vi "readDataArray.vi"(8 "error in (no error)":errorcluster, 10 "array":string[][](array[string]), 11 "Ao8FileReader in":refnum<class "Ao8FileReader.lvclass">) -> (0 "error out":errorcluster, 3 "Ao8FileReader out":refnum<class "Ao8FileReader.lvclass">)   [LabVIEW 2011, in "Tools.lvlib" / "Filing.lvlib" / "Ao8FileReader.lvclass"]
uses:
  Ao8FileReader.lvclass
  Ao8FileReader.lvclass/Ao8FileReader.ctl
  Hal/Channels/VoltOutput/AnalogOutput.lvclass
panel:
  out "channelAddresses":string[](array[string])
  out "Defaults":dbl[](array[numeric])
  out "data":dbl[][](array[numeric])
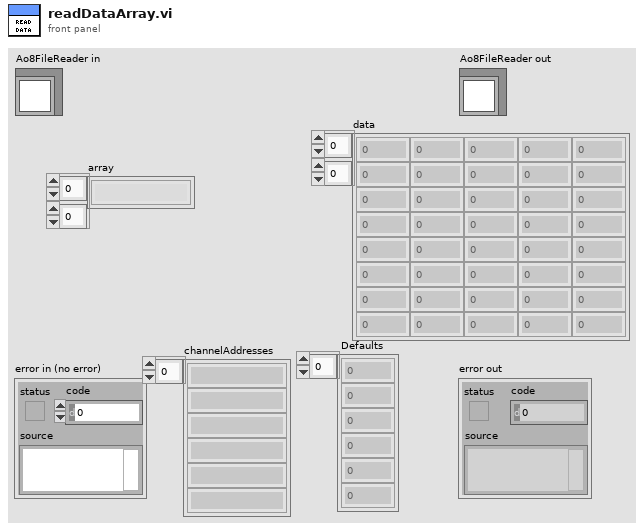
[diagram p1: front panel]
types:
  T1 = cluster{"Clock source":string, "Clock rate":dbl, "Start trigger line":string, "Sample Rate":dbl, "Sample No.":dbl}
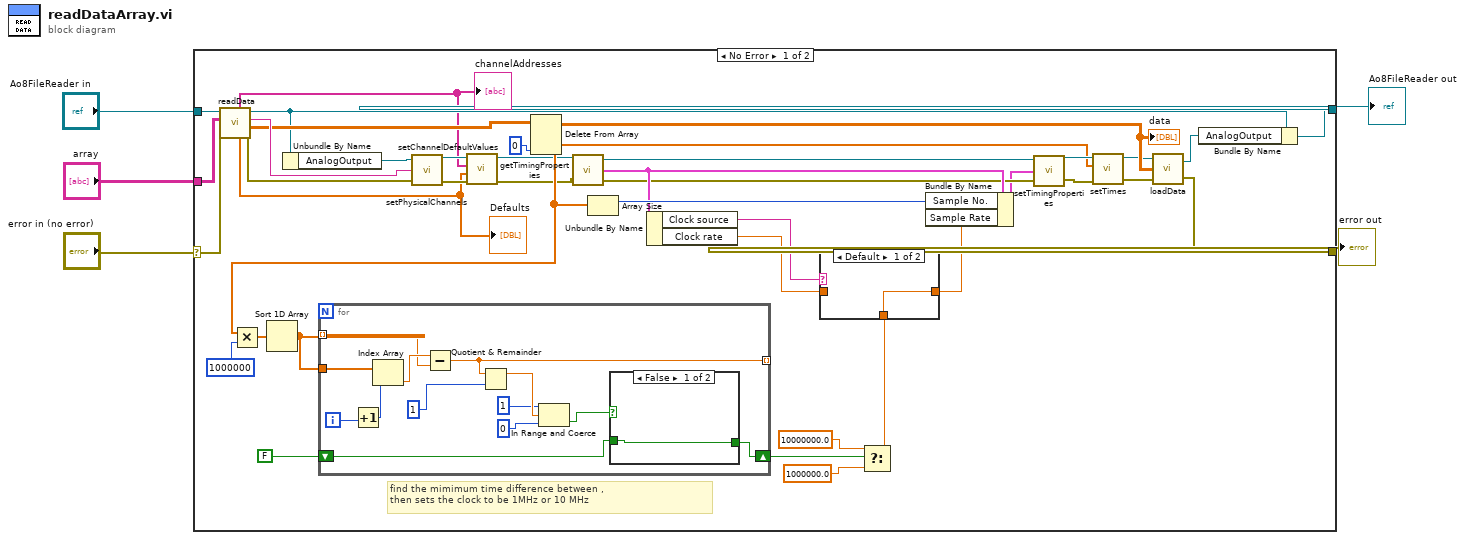
[diagram p0: block diagram]
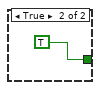
[diagram p3: hidden frame]
diagram:
  n1 = case shown="No Error" "error in (no error)" {
    selector: "error in (no error)" -> [w43 w63]
    tunnel: "Ao8FileReader in" -> [w45 w64]
    tunnel: "array" -> [w44 _]
    tunnel: [w13 w64] -> w3
    tunnel: [w16 w63] -> w2
    frame No Error {
      # "find the mimimum time difference between ,\nthen sets the clock to be 1MHz or 10 MHz"
      n2 = call-dynamic "readData.vi"("error in (no error)"=w43, "array"=w44, "FileReader in"=w45) -> ("error out"=w40:errorcluster, "Array"=w23:dbl[][], "channels"=w41:string, "FileReader out"=w15:refnum<class "Ao8FileReader.lvclass">, "Defaults"=w6:dbl[], "channelAddresses"=w7:string[])  [unwired: 3 in]
      "Defaults" <- w6
      "channelAddresses" <- w7
      n3 = Unbundle By Name(w15) -> ("AnalogOutput"=w42:refnum<class "AnalogOutput.lvclass">)
      n4 = call-dynamic "setPhysicalChannels.vi"("error in (no error)"=w40, "Physical Channels"=w41, "AnalogOutput.lvclass in"=w42) -> ("error out"=w10:errorcluster, "AnalogOutput.lvclass out"=w11:refnum<class "AnalogOutput.lvclass">)
      n5 = call "setChannelDefaultValues.vi"("error in (no error)"=w10, "calibratedValues"=w6, "channel_addresses"=w7, "AnalogOutput in"=w11) -> ("error out"=w9:errorcluster, "AnalogOutput out"=w8:refnum<class "AnalogOutput.lvclass">)  [unwired: 6 in]
      n6 = Delete From Array(array=w23, index (col)=0 ("disabled index (col)")) -> (deleted portion=w12:dbl[], array with subset deleted=w21:dbl[][])  [unwired: 2 in]
      "data" <- w21
      n7 = Multiply(x=w12, y=1000000) -> (x*y=w33:dbl[])
      n8 = Sort 1D Array(array=w33) -> (sorted array=w38:dbl[])
      n9 = for {
        tunnel: w38 -> [w56] mode=indexing
        tunnel: w38 -> [w60]
        tunnel: [w51] -> _ mode=indexing
        shift-right: [w48] -> w36
        shift-left: FALSE -> [w49]
        i -> [w59]
        n10 = Increment(x=w59) -> (x+1=w58:i32)
        n11 = Index Array(array=w60, index=w58) -> (element=w57:dbl)
        n12 = Subtract(x=w57, y=w56) -> (x-y=w51:dbl)
        n13 = Quotient & Remainder(x=w51, y=1) -> (x-y*floor(x/y)=w54:dbl)  [unwired: 1 out]
        n14 = In Range and Coerce(upper limit=1, x=w54, lower limit=0) -> (In Range?=w50:bool)  [unwired: 1 out]
        n15 = case shown="False" w50 {
          tunnel: w49 -> [w61 _]
          tunnel: [w61 TRUE] -> w48
          frame False {
          }
          frame True {
          }
        }
      }
      n16 = call "getTimingProperties.vi"("AnalogOutput.lvclass in"=w8, "error in (no error)"=w9) -> ("AnalogOutput.lvclass out"=w26:refnum<class "AnalogOutput.lvclass">, "Timing"=w31:T1, "error out"=w25:errorcluster)
      n17 = Array Size(array=w12) -> (size(s)=w39:i32)
      n18 = Unbundle By Name(w31) -> ("Clock source"=w30:string, "Clock rate"=w28:dbl)
      n19 = Select(t=10000000.0, s=w36, f=1000000.0) -> (s? t:f=w29:dbl)
      n20 = case shown="Default" w30 {
        tunnel: w29 -> [w46 _]
        tunnel: w28 -> [_ w47]
        tunnel: [w46 w47] -> w27
        frame Default {
        }
        frame "internal", "none" {
        }
      }
      n21 = Bundle By Name(cluster=w31, "Sample No."=w39, "Sample Rate"=w27) -> (w24:T1)
      n22 = call "setTimingProperties.vi"("error in (no error)"=w25, "Timing"=w24, "AnalogOutput.lvclass in"=w26) -> ("error out"=w18:errorcluster, "AnalogOutput.lvclass out"=w20:refnum<class "AnalogOutput.lvclass">)
      n23 = call "setTimes.vi"("error in (no error)"=w18, "times"=w12, "AnalogOutput in"=w20) -> ("error out"=w17:errorcluster, "AnalogOutput out"=w19:refnum<class "AnalogOutput.lvclass">)  [unwired: 7 in]
      n24 = call-dynamic "loadData.vi"("error in (no error)"=w17, "Data"=w21, "AnalogOutput in"=w19) -> ("error out"=w16:errorcluster, "AnalogOutput out"=w14:refnum<class "AnalogOutput.lvclass">)
      n25 = Bundle By Name(cluster=w15, "AnalogOutput"=w14) -> (w13:refnum<class "Ao8FileReader.lvclass">)
    }
    frame Error {
    }
  }
  "error out" <- w2
  "Ao8FileReader out" <- w3
